vi "new velocities.vi"(10 "Matriz m \nesperada":T1, 11 "m sem\ndeslizamento":T1) -> (2 "<m_o,m_c>":dbl format="%.2f", 3 "m sem \ndeslizamento \ne no \nsentido \noriginal":dbl[](array[numeric]), 4 "error":i32)   [LabVIEW 2018]
uses:
  <vilib>/Analysis/Matrix/Datatypes/RealMatrix.ctl
  <vilib>/Analysis/_algsub.llb/Real Vector Norm.vi
  <vilib>/Analysis/baseanly.llb/Real Dot Product.vi
  <vilib>/Analysis/NI_AALBase.lvlib
  <vilib>/Analysis/NI_AALPro.lvlib
  <vilib>/Analysis/Matrix/NI_Matrix.lvlib
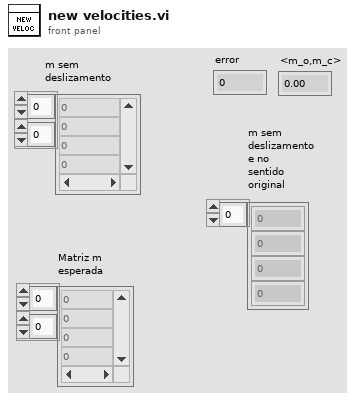
[diagram p1: front panel]
types:
  T1 = typedef "NI_Matrix.lvlib/RealMatrix.ctl" = dbl[][]
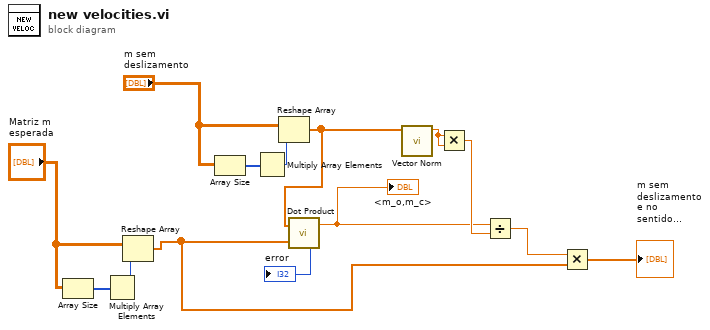
[diagram p0: block diagram]
diagram:
  n1 = Array Size(array="Matriz m \nesperada") -> (size(s)=w12:i32[])
  n2 = Multiply Array Elements(1:w12) -> (0:w11:i32)
  n3 = Reshape Array("Matriz m \nesperada", w11) -> (w9:dbl[])
  n4 = Array Size(array="m sem\ndeslizamento") -> (size(s)=w14:i32[])
  n5 = Multiply Array Elements(1:w14) -> (0:w13:i32)
  n6 = Reshape Array("m sem\ndeslizamento", w13) -> (w3:dbl[])
  n7 = call-poly <vilib>:"Dot Product.vi"("Y Vector"=w9, "X Vector"=w3) -> ("error"=→"error":i32, "X * Y"=w5:dbl)
  "<m_o,m_c>" <- w5
  n8 = call-poly <vilib>:"Vector Norm.vi"("Input Vector"=w3) -> ("norm"=w7:dbl)  [unwired: 9 in, 1 out]
  n9 = Multiply(x=w7, y=w7) -> (x*y=w6:dbl)
  n10 = Divide(x=w5, y=w6) -> (x/y=w4:dbl)
  n11 = Multiply(x=w4, y=w9) -> (x*y=→"m sem \ndeslizamento \ne no \nsentido \noriginal":dbl[])
